vi "3.7.vi"() -> ()   [LabVIEW 2014]
panel:
  out "Square Root":dbl
  in  "Number":dbl
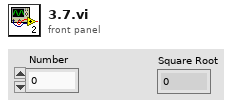
[diagram p1: front panel]
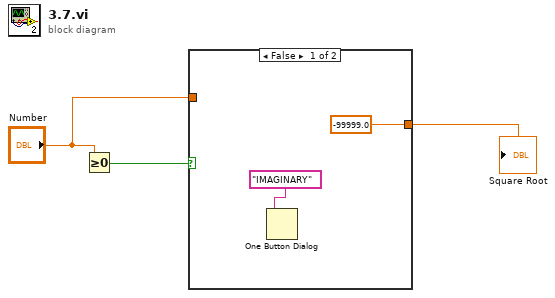
[diagram p0: block diagram]
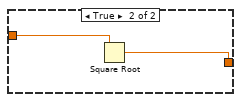
[diagram p2: hidden frame]
diagram:
  n1 = Greater Or Equal To 0?(x="Number") -> (x >= 0?=w1:bool)
  n2 = case shown="False" w1 {
    tunnel: [-99999.0 w6] -> w3
    tunnel: "Number" -> [_ w7]
    frame False {
      n3 = One Button Dialog(message="IMAGINARY") -> ()  [unwired: 1 in, 1 out]
    }
    frame True {
      n4 = Square Root(x=w7) -> (sqrt(x)=w6:dbl)
    }
  }
  "Square Root" <- w3
